vi "ME79ConfigLoadAndSave.vi"(6 "Freq List file":path, 7 "Freq List In":cluster{"Freq":dbl, "Amp":dbl}[](array[cluster]), 8 "error in (no error)":errorcluster, 9 "Config In":T1={"PSU"={"Current Lower (mA)"=0.0, "Current Upper (mA)"=0.0, "Voltage Lower (V)"=0.0, "Voltage Upper (V)"=0.0}, "Mic"={"Sensitivity (mV/Pa)"={"Lower"=0.0, "Upper"=0.0}, "THD (%)"={"Lower"=0.0, "Upper"=0.0}, "Freq Response"=[]}, "Power Supply"={"Channel Name"="1", "Source Delay (Sec)"=0.5, "Measurement:Sense"=1008, "voltage level"=0.0, "voltage level range"=20.0, "current limit"=0.02, "current limit range"=0.02, "resource name"="PSU"}, "Test Sweep"={"Input Settings"={"IEPE min time to settle [s]"=0.0, "Responce Channel Settings"={"DSA response channel settings"={"coupling"=10045, "enable IEPE excitation"=FALSE, "IEPE current [mA]"=4.0}, "response channel info"={"sensor sensitivity"=1000.0, "engineering units"=1, "dB reference"=1.0, "custom label"="EU", "weighting filter"=0, "pregain"=0.0}, "AI response settings"={"response channel"="SOUNDACQ/ai1", "max value [V]"=10.0, "min value [V]"=-10.0, "terminal configuration"=-1}}, "Stimulus Channel Settings"={"AI stimulus settings"={"stimulus channel"="SOUNDACQ/ai0", "max value [V]"=2.0, "min value [V]"=-2.0, "terminal configuration"=-1}, "DSA stimulus channel settings"={"coupling"=10045, "enable IEPE excitation"=TRUE, "IEPE current [mA]"=4.0}, "stimulus channel info"={"sensor sensitivity"=11.4, "engineering units"=2, "dB reference"=2e-05, "custom label"="EU", "weighting filter"=0, "pregain"=0.0}}}, "Output Settings"={"AO source settings"={"excitation channel"="SOUNDACQ/ao0", "max value [V]"=10.0, "min value [V]"=-10.0, "terminal configuration"=-1}}}} {"Test Sweep"."Output Settings"."AO source settings"."terminal configuration" items=["Default"=-1, "RSE"=10083, "Differential"=10106, "Pseudodifferential"=12529]; "Test Sweep"."Output Settings"."AO source settings"."min value [V]" format="%0.2f"; "Test Sweep"."Output Settings"."AO source settings"."max value [V]" format="%0.2f"; "Test Sweep"."Input Settings"."Stimulus Channel Settings"."stimulus channel info"."pregain" format="%.2f"; "Test Sweep"."Input Settings"."Stimulus Channel Settings"."stimulus channel info"."weighting filter" items=["Linear", "A-weighting", "B-weighting", "C-weighting", "ITU-R 468-4", "Dolby", "CCITT", "C-message", "Wb", "Wc", "Wd", "We", "Wf", "Wh", "Wj", "Wk", "Wm", "AES17 20 kHz lowpass", "AES17 40 kHz lowpass", "AES17 20 kHz highpass", "AES17 40 kHz highpass"]; "Test Sweep"."Input Settings"."Stimulus Channel Settings"."stimulus channel info"."dB reference" format="%^.1e"; "Test Sweep"."Input Settings"."Stimulus Channel Settings"."stimulus channel info"."engineering units" items=["custom..."=0, "V"=1, "A"=21, "C"=30, "pC"=31, "s"=32, "-"=29, "Pa"=2, "N"=20, "g"=3, "m/s^2"=4, "m/s"=5, "m"=6, "mm/s"=12, "mm"=13, "micron/s"=14, "micron"=15, "in/s^2"=7, "in/s"=8, "in"=9, "mil/s"=10, "mil"=11, "rad/s^2"=16, "rad/s"=17, "rad"=18, "deg/s^2"=26, "deg/s"=27, "deg"=28, "RPM"=22, "cycle/s^2"=23, "Hz"=24, "cycle"=25, "strain"=19]; "Test Sweep"."Input Settings"."Stimulus Channel Settings"."stimulus channel info"."sensor sensitivity" format="%#_5f"; "Test Sweep"."Input Settings"."Stimulus Channel Settings"."DSA stimulus channel settings"."IEPE current [mA]" format="%.1f"; "Test Sweep"."Input Settings"."Stimulus Channel Settings"."DSA stimulus channel settings"."coupling" items=["AC"=10045, "DC"=10050, "GND"=10066]; "Test Sweep"."Input Settings"."Stimulus Channel Settings"."AI stimulus settings"."terminal configuration" items=["Default"=-1, "RSE"=10083, "NRSE"=10078, "Differential"=10106, "Pseudodifferential"=12529]; "Test Sweep"."Input Settings"."Stimulus Channel Settings"."AI stimulus settings"."min value [V]" format="%.2f"; "Test Sweep"."Input Settings"."Stimulus Channel Settings"."AI stimulus settings"."max value [V]" format="%.2f"; "Test Sweep"."Input Settings"."Responce Channel Settings"."AI response settings"."terminal configuration" items=["Default"=-1, "RSE"=10083, "NRSE"=10078, "Differential"=10106, "Pseudodifferential"=12529]; "Test Sweep"."Input Settings"."Responce Channel Settings"."AI response settings"."min value [V]" format="%.2f"; "Test Sweep"."Input Settings"."Responce Channel Settings"."AI response settings"."max value [V]" format="%.2f"; "Test Sweep"."Input Settings"."Responce Channel Settings"."response channel info"."pregain" format="%.2f"; "Test Sweep"."Input Settings"."Responce Channel Settings"."response channel info"."weighting filter" items=["Linear", "A-weighting", "B-weighting", "C-weighting", "ITU-R 468-4", "Dolby", "CCITT", "C-message", "Wb", "Wc", "Wd", "We", "Wf", "Wh", "Wj", "Wk", "Wm", "AES17 20 kHz lowpass", "AES17 40 kHz lowpass", "AES17 20 kHz highpass", "AES17 40 kHz highpass"]; "Test Sweep"."Input Settings"."Responce Channel Settings"."response channel info"."dB reference" format="%^.1e"; "Test Sweep"."Input Settings"."Responce Channel Settings"."response channel info"."engineering units" items=["custom..."=0, "V"=1, "A"=21, "C"=30, "pC"=31, "s"=32, "-"=29, "Pa"=2, "N"=20, "g"=3, "m/s^2"=4, "m/s"=5, "m"=6, "mm/s"=12, "mm"=13, "micron/s"=14, "micron"=15, "in/s^2"=7, "in/s"=8, "in"=9, "mil/s"=10, "mil"=11, "rad/s^2"=16, "rad/s"=17, "rad"=18, "deg/s^2"=26, "deg/s"=27, "deg"=28, "RPM"=22, "cycle/s^2"=23, "Hz"=24, "cycle"=25, "strain"=19]; "Test Sweep"."Input Settings"."Responce Channel Settings"."response channel info"."sensor sensitivity" format="%#_5f"; "Test Sweep"."Input Settings"."Responce Channel Settings"."DSA response channel settings"."IEPE current [mA]" format="%.1f"; "Test Sweep"."Input Settings"."Responce Channel Settings"."DSA response channel settings"."coupling" items=["AC"=10045, "DC"=10050, "GND"=10066]; "Test Sweep"."Input Settings"."IEPE min time to settle [s]" format="%.1f"; "Power Supply"."current limit range" format="%_6p"; "Power Supply"."current limit" format="%_6p"; "Power Supply"."voltage level range" format="%_6p"; "Power Supply"."voltage level" format="%_6p"; "Power Supply"."Measurement:Sense" items=["Local"=1008, "Remote"=1009]; "Power Supply"."Source Delay (Sec)" format="%_6p"}, 10 "Mode (F-Read)":bool, 11 "Config file":path) -> (0 "error out":errorcluster, 2 "Config Out":T1={"PSU"={"Current Lower (mA)"=0.0, "Current Upper (mA)"=0.0, "Voltage Lower (V)"=0.0, "Voltage Upper (V)"=0.0}, "Mic"={"Sensitivity (mV/Pa)"={"Lower"=0.0, "Upper"=0.0}, "THD (%)"={"Lower"=0.0, "Upper"=0.0}, "Freq Response"=[]}, "Power Supply"={"Channel Name"="1", "Source Delay (Sec)"=0.5, "Measurement:Sense"=1008, "voltage level"=0.0, "voltage level range"=20.0, "current limit"=0.02, "current limit range"=0.02, "resource name"="PSU"}, "Test Sweep"={"Input Settings"={"IEPE min time to settle [s]"=0.0, "Responce Channel Settings"={"DSA response channel settings"={"coupling"=10045, "enable IEPE excitation"=FALSE, "IEPE current [mA]"=4.0}, "response channel info"={"sensor sensitivity"=1000.0, "engineering units"=1, "dB reference"=1.0, "custom label"="EU", "weighting filter"=0, "pregain"=0.0}, "AI response settings"={"response channel"="SOUNDACQ/ai1", "max value [V]"=10.0, "min value [V]"=-10.0, "terminal configuration"=-1}}, "Stimulus Channel Settings"={"AI stimulus settings"={"stimulus channel"="SOUNDACQ/ai0", "max value [V]"=2.0, "min value [V]"=-2.0, "terminal configuration"=-1}, "DSA stimulus channel settings"={"coupling"=10045, "enable IEPE excitation"=TRUE, "IEPE current [mA]"=4.0}, "stimulus channel info"={"sensor sensitivity"=11.4, "engineering units"=2, "dB reference"=2e-05, "custom label"="EU", "weighting filter"=0, "pregain"=0.0}}}, "Output Settings"={"AO source settings"={"excitation channel"="SOUNDACQ/ao0", "max value [V]"=10.0, "min value [V]"=-10.0, "terminal configuration"=-1}}}} {"Test Sweep"."Output Settings"."AO source settings"."terminal configuration" items=["Default"=-1, "RSE"=10083, "Differential"=10106, "Pseudodifferential"=12529]; "Test Sweep"."Output Settings"."AO source settings"."min value [V]" format="%0.2f"; "Test Sweep"."Output Settings"."AO source settings"."max value [V]" format="%0.2f"; "Test Sweep"."Input Settings"."Stimulus Channel Settings"."stimulus channel info"."pregain" format="%.2f"; "Test Sweep"."Input Settings"."Stimulus Channel Settings"."stimulus channel info"."weighting filter" items=["Linear", "A-weighting", "B-weighting", "C-weighting", "ITU-R 468-4", "Dolby", "CCITT", "C-message", "Wb", "Wc", "Wd", "We", "Wf", "Wh", "Wj", "Wk", "Wm", "AES17 20 kHz lowpass", "AES17 40 kHz lowpass", "AES17 20 kHz highpass", "AES17 40 kHz highpass"]; "Test Sweep"."Input Settings"."Stimulus Channel Settings"."stimulus channel info"."dB reference" format="%^.1e"; "Test Sweep"."Input Settings"."Stimulus Channel Settings"."stimulus channel info"."engineering units" items=["custom..."=0, "V"=1, "A"=21, "C"=30, "pC"=31, "s"=32, "-"=29, "Pa"=2, "N"=20, "g"=3, "m/s^2"=4, "m/s"=5, "m"=6, "mm/s"=12, "mm"=13, "micron/s"=14, "micron"=15, "in/s^2"=7, "in/s"=8, "in"=9, "mil/s"=10, "mil"=11, "rad/s^2"=16, "rad/s"=17, "rad"=18, "deg/s^2"=26, "deg/s"=27, "deg"=28, "RPM"=22, "cycle/s^2"=23, "Hz"=24, "cycle"=25, "strain"=19]; "Test Sweep"."Input Settings"."Stimulus Channel Settings"."stimulus channel info"."sensor sensitivity" format="%#_5f"; "Test Sweep"."Input Settings"."Stimulus Channel Settings"."DSA stimulus channel settings"."IEPE current [mA]" format="%.1f"; "Test Sweep"."Input Settings"."Stimulus Channel Settings"."DSA stimulus channel settings"."coupling" items=["AC"=10045, "DC"=10050, "GND"=10066]; "Test Sweep"."Input Settings"."Stimulus Channel Settings"."AI stimulus settings"."terminal configuration" items=["Default"=-1, "RSE"=10083, "NRSE"=10078, "Differential"=10106, "Pseudodifferential"=12529]; "Test Sweep"."Input Settings"."Stimulus Channel Settings"."AI stimulus settings"."min value [V]" format="%.2f"; "Test Sweep"."Input Settings"."Stimulus Channel Settings"."AI stimulus settings"."max value [V]" format="%.2f"; "Test Sweep"."Input Settings"."Responce Channel Settings"."AI response settings"."terminal configuration" items=["Default"=-1, "RSE"=10083, "NRSE"=10078, "Differential"=10106, "Pseudodifferential"=12529]; "Test Sweep"."Input Settings"."Responce Channel Settings"."AI response settings"."min value [V]" format="%.2f"; "Test Sweep"."Input Settings"."Responce Channel Settings"."AI response settings"."max value [V]" format="%.2f"; "Test Sweep"."Input Settings"."Responce Channel Settings"."response channel info"."pregain" format="%.2f"; "Test Sweep"."Input Settings"."Responce Channel Settings"."response channel info"."weighting filter" items=["Linear", "A-weighting", "B-weighting", "C-weighting", "ITU-R 468-4", "Dolby", "CCITT", "C-message", "Wb", "Wc", "Wd", "We", "Wf", "Wh", "Wj", "Wk", "Wm", "AES17 20 kHz lowpass", "AES17 40 kHz lowpass", "AES17 20 kHz highpass", "AES17 40 kHz highpass"]; "Test Sweep"."Input Settings"."Responce Channel Settings"."response channel info"."dB reference" format="%^.1e"; "Test Sweep"."Input Settings"."Responce Channel Settings"."response channel info"."engineering units" items=["custom..."=0, "V"=1, "A"=21, "C"=30, "pC"=31, "s"=32, "-"=29, "Pa"=2, "N"=20, "g"=3, "m/s^2"=4, "m/s"=5, "m"=6, "mm/s"=12, "mm"=13, "micron/s"=14, "micron"=15, "in/s^2"=7, "in/s"=8, "in"=9, "mil/s"=10, "mil"=11, "rad/s^2"=16, "rad/s"=17, "rad"=18, "deg/s^2"=26, "deg/s"=27, "deg"=28, "RPM"=22, "cycle/s^2"=23, "Hz"=24, "cycle"=25, "strain"=19]; "Test Sweep"."Input Settings"."Responce Channel Settings"."response channel info"."sensor sensitivity" format="%#_5f"; "Test Sweep"."Input Settings"."Responce Channel Settings"."DSA response channel settings"."IEPE current [mA]" format="%.1f"; "Test Sweep"."Input Settings"."Responce Channel Settings"."DSA response channel settings"."coupling" items=["AC"=10045, "DC"=10050, "GND"=10066]; "Test Sweep"."Input Settings"."IEPE min time to settle [s]" format="%.1f"; "Power Supply"."current limit range" format="%_6p"; "Power Supply"."current limit" format="%_6p"; "Power Supply"."voltage level range" format="%_6p"; "Power Supply"."voltage level" format="%_6p"; "Power Supply"."Measurement:Sense" items=["Local"=1008, "Remote"=1009]; "Power Supply"."Source Delay (Sec)" format="%_6p"}, 3 "Freq List Out":cluster{"Freq":dbl, "Amp":dbl}[](array[cluster]))   [LabVIEW 2018]
uses:
  Types/ME79 Specs.ctl
  <vilib>/addons/_NISVFA/_Shared subVIs/Controls/svc_DSA Channel Settings.ctl
  <vilib>/addons/_NISVFA/_Shared subVIs/Controls/svc_Channel Info.ctl
  <vilib>/addons/_NISVFA/_Shared subVIs/Controls/svc_Engineering Units Text Ring.ctl
  <vilib>/addons/_NISVFA/_Shared subVIs/Controls/svc_Weighting Filter Text Ring.ctl
  <vilib>/Utility/file.llb/Read Delimited Spreadsheet (DBL).vi
  <vilib>/Utility/xml.llb/Read From XML File(string).vi
  <vilib>/Utility/file.llb/Write Delimited Spreadsheet (DBL).vi
  <vilib>/Utility/xml.llb/Write to XML File(string).vi
panel:
  # "Power Supply"
  # "Power Supply"
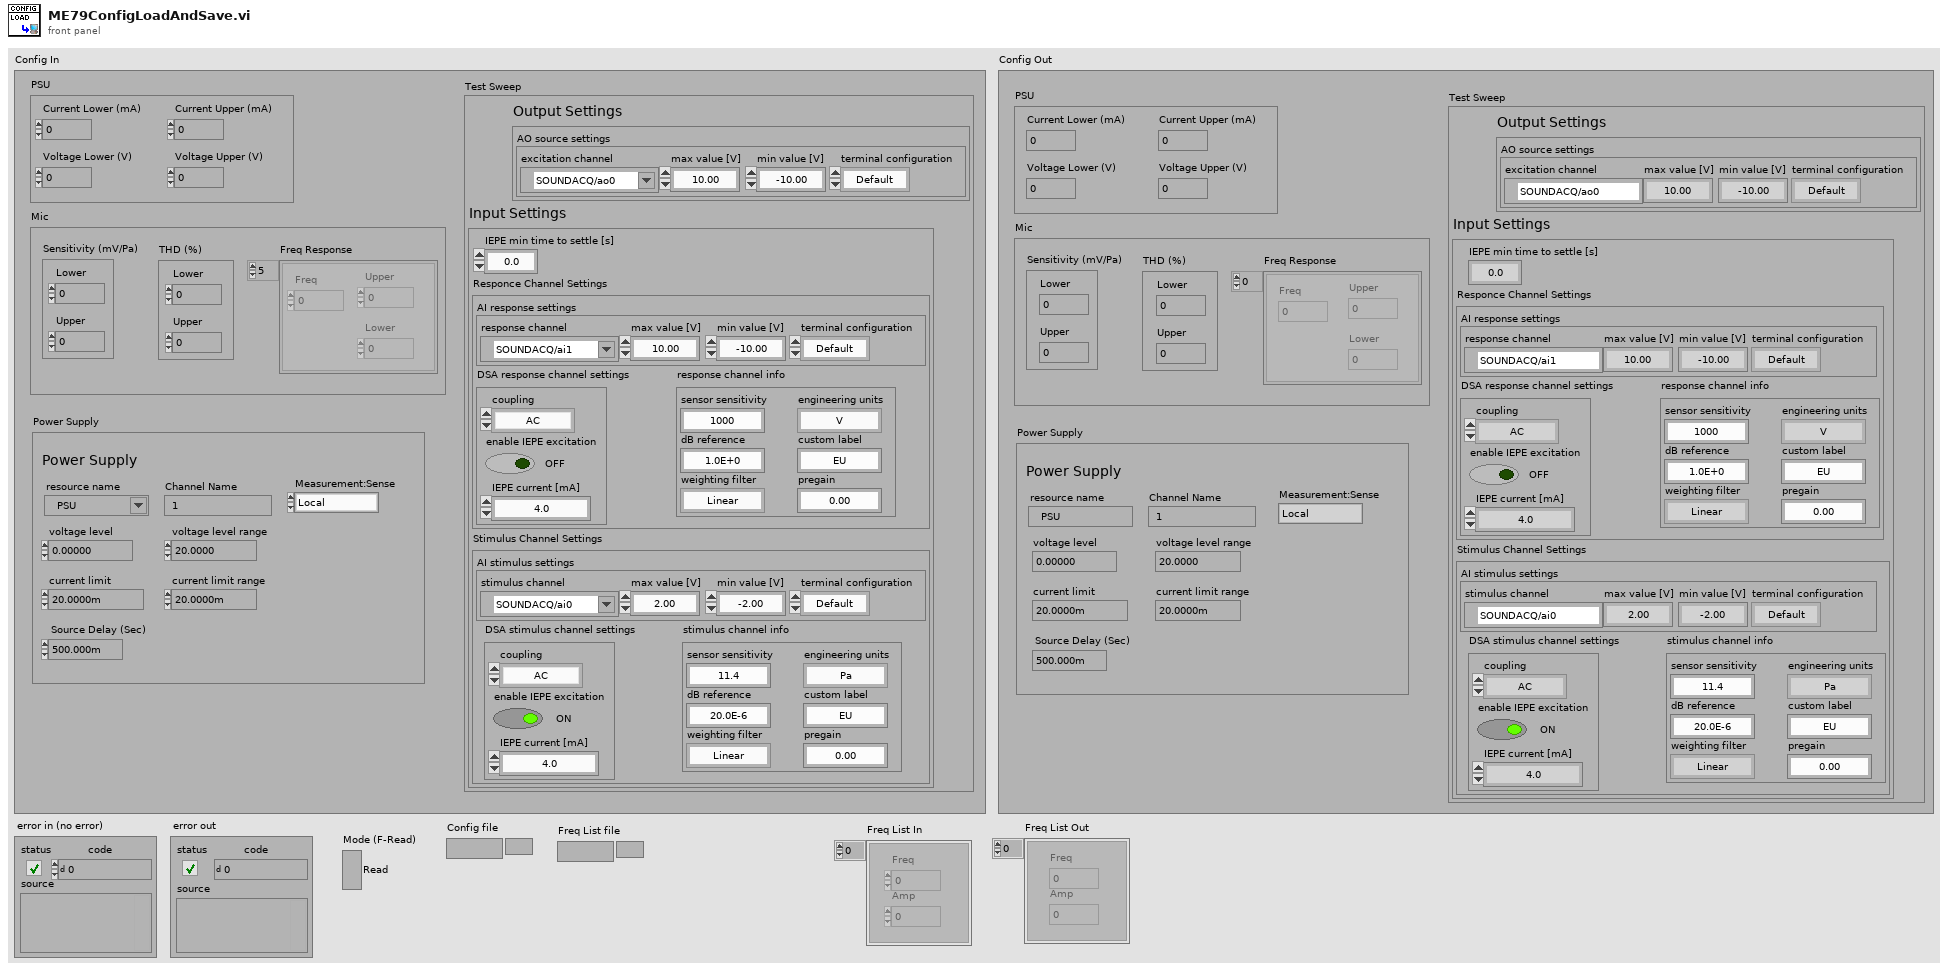
[diagram p1: front panel]
types:
  T1 = typedef "ME79 Specs.ctl" = cluster{"PSU":cluster{"Current Lower (mA)":dbl, "Current Upper (mA)":dbl, "Voltage Lower (V)":dbl, "Voltage Upper (V)":dbl}, "Mic":cluster{"Sensitivity (mV/Pa)":cluster{"Lower":dbl, "Upper":dbl}, "THD (%)":cluster{"Lower":dbl, "Upper":dbl}, "Freq Response":cluster{"Freq":dbl, "Upper":dbl, "Lower":dbl}[]}, "Power Supply":cluster{"Channel Name":string, "Source Delay (Sec)":dbl, "Measurement:Sense":i32, "voltage level":dbl, "voltage level range":dbl, "current limit":dbl, "current limit range":dbl, "resource name":refnum<k15>}, "Test Sweep":cluster{"Input Settings":cluster{"IEPE min time to settle [s]":dbl, "Responce Channel Settings":cluster{"DSA response channel settings":T2, "response channel info":T3, "AI response settings":cluster{"response channel":tag, "max value [V]":dbl, "min value [V]":dbl, "terminal configuration":i32}}, "Stimulus Channel Settings":cluster{"AI stimulus settings":cluster{"stimulus channel":tag, "max value [V]":dbl, "min value [V]":dbl, "terminal configuration":i32}, "DSA stimulus channel settings":T2, "stimulus channel info":T3}}, "Output Settings":cluster{"AO source settings":cluster{"excitation channel":tag, "max value [V]":dbl, "min value [V]":dbl, "terminal configuration":i32}}}}
  T2 = typedef "svc_DSA Channel Settings.ctl" = cluster{"coupling":i32, "enable IEPE excitation":bool, "IEPE current [mA]":dbl}
  T3 = typedef "svc_Channel Info.ctl" = cluster{"sensor sensitivity":dbl, "engineering units":T4, "dB reference":dbl, "custom label":string, "weighting filter":T5, "pregain":dbl}
  T4 = typedef "svc_Engineering Units Text Ring.ctl" = u16
  T5 = typedef "svc_Weighting Filter Text Ring.ctl" = u16
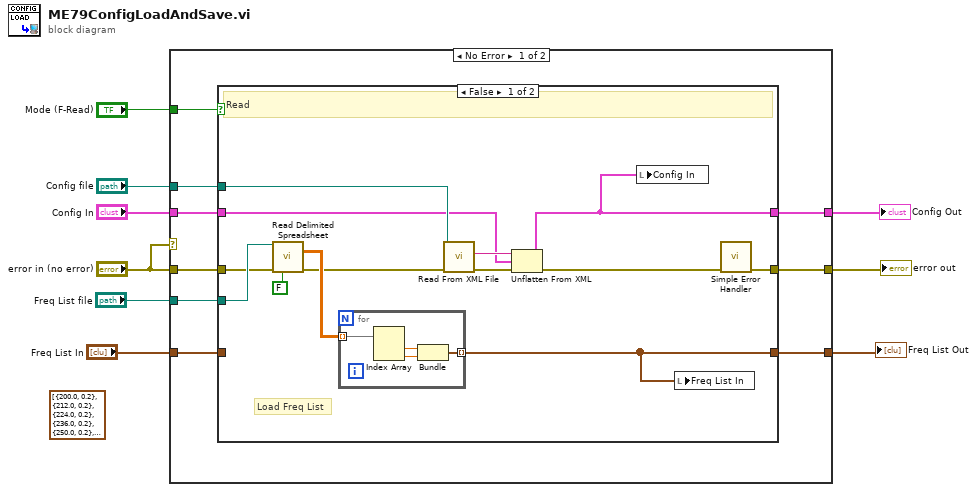
[diagram p0: block diagram]
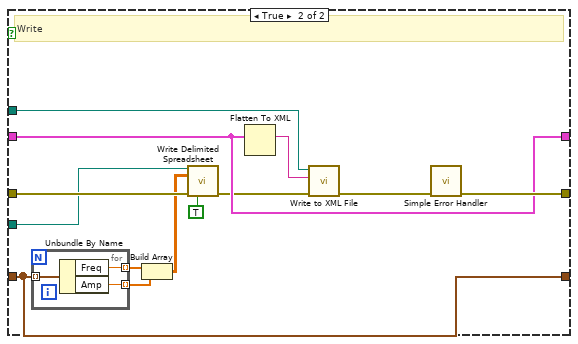
[diagram p2: hidden frame]
diagram:
  (unwired) cluster{"Freq":dbl, "Amp":dbl}[] [{"Freq"=200.0, "Amp"=0.2}, {"Freq"=212.0, "Amp"=0.2}, {"Freq"=224.0, "Amp"=0.2}, {"Freq"=236.0, "Amp"=0.2}, {"Freq"=250.0, "Amp"=0.2}, {"Freq"=265.0, "Amp"=0.2}, {"Freq"=280.0, "Amp"=0.2}, {"Freq"=300.0, "Amp"=0.2}, {"Freq"=315.0, "Amp"=0.2}, {"Freq"=335.0, "Amp"=0.2}, {"Freq"=355.0, "Amp"=0.2}, {"Freq"=375.0, "Amp"=0.2}, {"Freq"=400.0, "Amp"=0.2}, {"Freq"=425.0, "Amp"=0.2}, {"Freq"=450.0, "Amp"=0.2}, {"Freq"=475.0, "Amp"=0.2}, {"Freq"=500.0, "Amp"=0.2}, {"Freq"=530.0, "Amp"=0.2}, {"Freq"=560.0, "Amp"=0.2}, {"Freq"=600.0, "Amp"=0.2}, {"Freq"=630.0, "Amp"=0.2}, {"Freq"=670.0, "Amp"=0.2}, {"Freq"=710.0, "Amp"=0.2}, {"Freq"=750.0, "Amp"=0.2}, {"Freq"=800.0, "Amp"=0.2}, {"Freq"=850.0, "Amp"=0.2}, {"Freq"=900.0, "Amp"=0.2}, {"Freq"=950.0, "Amp"=0.2}, {"Freq"=1000.0, "Amp"=0.2}, {"Freq"=1060.0, "Amp"=0.2}, {"Freq"=1120.0, "Amp"=0.2}, {"Freq"=1180.0, "Amp"=0.2}, {"Freq"=1250.0, "Amp"=0.2}, {"Freq"=1320.0, "Amp"=0.2}, {"Freq"=1400.0, "Amp"=0.2}, {"Freq"=1500.0, "Amp"=0.2}, {"Freq"=1600.0, "Amp"=0.2}, {"Freq"=1700.0, "Amp"=0.2}, {"Freq"=1800.0, "Amp"=0.2}, {"Freq"=1900.0, "Amp"=0.2}, {"Freq"=2000.0, "Amp"=0.2}, {"Freq"=2120.0, "Amp"=0.2}, {"Freq"=2240.0, "Amp"=0.2}, {"Freq"=2360.0, "Amp"=0.2}, {"Freq"=2500.0, "Amp"=0.2}, {"Freq"=2650.0, "Amp"=0.2}, {"Freq"=2800.0, "Amp"=0.2}, {"Freq"=3000.0, "Amp"=0.2}, {"Freq"=3150.0, "Amp"=0.2}, {"Freq"=3350.0, "Amp"=0.2}, {"Freq"=3550.0, "Amp"=0.2}, {"Freq"=3750.0, "Amp"=0.2}, {"Freq"=4000.0, "Amp"=0.2}, {"Freq"=4250.0, "Amp"=0.2}, {"Freq"=4500.0, "Amp"=0.2}, {"Freq"=4750.0, "Amp"=0.2}, {"Freq"=5000.0, "Amp"=0.2}, {"Freq"=5300.0, "Amp"=0.2}, {"Freq"=5600.0, "Amp"=0.2}, {"Freq"=6000.0, "Amp"=0.2}, {"Freq"=6300.0, "Amp"=0.2}, {"Freq"=6700.0, "Amp"=0.2}, {"Freq"=7100.0, "Amp"=0.2}, {"Freq"=7500.0, "Amp"=0.2}, {"Freq"=8000.0, "Amp"=0.2}] ("Freq List Out")
  n1 = case shown="No Error" "error in (no error)" {
    tunnel: "Mode (F-Read)" -> [w18 _]
    tunnel: "Config file" -> [w17 _]
    tunnel: "Config In" -> [w16 w53]
    tunnel: "error in (no error)" -> [w15 w54]
    tunnel: [w14 w54] -> w5
    tunnel: [w13 w53] -> w4
    tunnel: "Freq List file" -> [w12 _]
    tunnel: "Freq List In" -> [w11 w52]
    tunnel: [w10 w52] -> w2
    frame No Error {
      n2 = case shown="False" w18 {
        tunnel: w17 -> [w31 w47]
        tunnel: w16 -> [w29 w45]
        tunnel: w15 -> [w25 w41]
        tunnel: [w27 w46] -> w14
        tunnel: [w19 w45] -> w13
        tunnel: w12 -> [w26 w40]
        tunnel: w11 -> [_ w36]
        tunnel: [w20 w36] -> w10
        frame False {
          # "Load Freq List"
          # "Read"
          n3 = call-poly <vilib>:"Read Delimited Spreadsheet.vi"("file path (dialog if empty)"=w26, "error in (no error)"=w25, "transpose? (F)"=FALSE) -> ("all rows"=w23:dbl[][], "error out"=w22:errorcluster)  [unwired: 7 in, 4 out]
          n4 = for {
            tunnel: w23 -> [w35] mode=indexing
            tunnel: [w32] -> w20 mode=indexing
            n5 = Index Array(array=w35) -> (element #1=w34:dbl, element #2=w33:dbl)  [unwired: 2 in]
            n6 = Bundle("Numeric"=w34, "Numeric"=w33) -> (w32:cluster{"Numeric":dbl, "Numeric":dbl})  [unwired: 1 in]
          }
          n7 = call-poly <vilib>:"Read From XML File.vi"("error in (no error)"=w22, "XML File Path"=w31) -> ("error out"=w28:errorcluster, "XML Elements"=w30:string)  [unwired: 7 in, 1 out]
          n8 = Unflatten From XML(xml string=w30, type=w29, error in (no error)=w28) -> (value=w19:T1, error out=w21:errorcluster)
          n9 = local write "Config In"(w19) -> ()
          n10 = local write "Freq List In"(w20) -> ()
          n11 = call <vilib>:"Simple Error Handler.vi"("error in (no error)"=w21) -> ("error out"=w27:errorcluster)  [unwired: 4 in, 4 out]
        }
        frame True {
          # "Write"
          n12 = for {
            tunnel: w36 -> [w51] mode=indexing
            tunnel: [w50] -> w43 mode=indexing
            tunnel: [w49] -> w42 mode=indexing
            n13 = Unbundle By Name(w51) -> ("Freq"=w50:dbl, "Amp"=w49:dbl)
          }
          n14 = Build Array(w43, w42) -> (w39:dbl[][])
          n15 = call-poly <vilib>:"Write Delimited Spreadsheet.vi"("file path (dialog if empty)"=w40, "2D data"=w39, "error in (no error)"=w41, "transpose? (no:F)"=TRUE) -> ("error out"=w37:errorcluster)  [unwired: 10 in, 1 out]
          n16 = Flatten To XML(anything=w45) -> (xml string=w48:string)
          n17 = call-poly <vilib>:"Write to XML File.vi"("error in (no error)"=w37, "XML Input"=w48, "XML File Path"=w47) -> ("error out"=w44:errorcluster)  [unwired: 6 in, 2 out]
          n18 = call <vilib>:"Simple Error Handler.vi"("error in (no error)"=w44) -> ("error out"=w46:errorcluster)  [unwired: 4 in, 4 out]
        }
      }
    }
    frame Error {
    }
  }
  "error out" <- w5
  "Config Out" <- w4
  "Freq List Out" <- w2
